vi "ConfigureRotatorPoint.vi"(10 "Rotator Position Min":dbl, 11 "Rotator Position Max":dbl) -> ()   [LabVIEW 2025]
doc: "Author: Scott Hannahs <sth@magnet.fsu.edu>\n\nThis software is licensed for use under the “MIT License\"\nCopyright (c) 2025 Scott Hannahs, sth@sth@magnet.sthnet.net\n\nPermission is hereby granted, free of charge, to any person obtaining a copy of this software and associated documentation files (the \"Software\"), to deal in the Software without restriction, including without limitation the rights to use, copy, modify, merge, publish, distribute, sublicense, and/or sell copies of the Software, and to permit persons to whom the Software is furnished to do so, subject to the following conditions: The above copyright notice and this permission notice shall be included in all copies or substantial portions of the Software.\n\nTHE SOFTWARE IS PROVIDED \"AS IS\", WITHOUT WARRANTY OF ANY KIND, EXPRESS OR IMPLIED, INCLUDING BUT NOT LIMITED TO THE WARRANTIES OF MERCHANTABILITY, FITNESS FOR A PARTICULAR PURPOSE AND NONINFRINGEMENT. IN NO EVENT SHALL THE AUTHORS OR COPYRIGHT HOLDERS BE LIABLE FOR ANY CLAIM, DAMAGES OR OTHER LIABILITY, WHETHER IN AN ACTION OF CONTRACT, TORT OR OTHERWISE, ARISING FROM, OUT OF OR IN CONNECTION WITH THE SOFTWARE OR THE USE OR OTHER DEALINGS IN THE SOFTWARE."
uses:
  Sub Controls/Instrument.ctl
  Sub Controls/NML GPIB List.ctl
panel:
  in  "Motor type":bool=TRUE
  out "Instrument":T1
  in  "Controls":refnum<vi>[](array[refnum])
  in  "GPIB Settings":T3 {"#16"."Parameters" format="%.3e"; "#20"."Parameters" format="%.3e"; "#18"."Parameters" format="%.3e"; "#17"."Parameters" format="%.3e"; "#19"."Parameters" format="%.3e"; "#11"."Parameters" format="%.3e"; "#15"."Parameters" format="%.3e"; "#13"."Parameters" format="%.3e"; "#12"."Parameters" format="%.3e"; "#14"."Parameters" format="%.3e"; "#6"."Parameters" format="%.3e"; "#10"."Parameters" format="%.3e"; "#8"."Parameters" format="%.3e"; "#7"."Parameters" format="%.3e"; "#9"."Parameters" format="%.3e"; "#1"."Parameters" format="%.3e"; "#5"."Parameters" format="%.3e"; "#3"."Parameters" format="%.3e"; "#2"."Parameters" format="%.3e"; "#4"."Parameters" format="%.3e"}
  in  "Done":bool
  # "BLM"
  # "IMS"
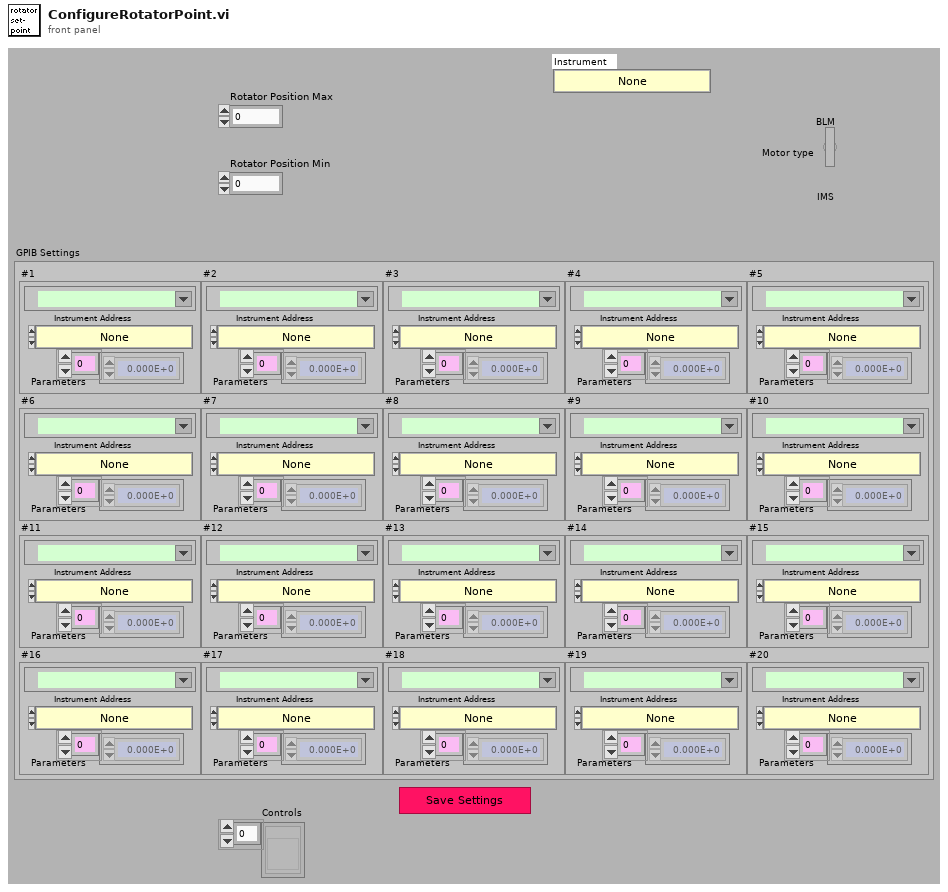
[diagram p1: front panel]
types:
  T1 = typedef "NML GPIB List.ctl" = enum16{"None", "Field", "Field - SCM1", "DMM", "DMM - HP 34401", "Keithley 2XXX", "Running DMM Ave", "Running HP34401", "Running K2XXX Ave", "SRS 830 - CH 1", "SRS 830 - CH1 & 2", "SRS PTC10", "Signal Rec 7265 - X", "Signal Rec 7265 - X&Y", "DRC 93C - Sample", "DRC 93C - Control", "DRC 93C - Sam&Con", "CryoCon Sensor A", "CryoCon Sensor B", "Cond 20C Sensor 1", "Cond 20C Sensor 2", "LS 336 Read", "LS 340 Read", "LS 370 Read", "LS 370 Select", "AVS 46 Bridge", "BLM Rotator Read Position", "Linear Research 700", "LR 700 Select", "Keithley 3330 - LCZ", "A-H Capacitance", "Digital Integrator", "SRS 400 Phot Ctr", "LakeShore VSM", "AMI He Level Meter", "Time Stamp", "Wait", "Invert Current", "K230 Linear V", "K230 VÅB^2", "Temp Ramp", "Power Ramp", "Freq Sweep", "LTC Stable T", "Scanner Step", "IMS Stepper Increment", "BLM Stepper Increment", "Omega CNi32"}
  T2 = typedef "Instrument.ctl" = cluster{"Instrument":T1, "Instrument Address":refnum<visa-resource-name>, "Parameters":dbl[]}
  T3 = cluster{"#1":T2, "#2":T2, "#3":T2, "#4":T2, "#5":T2, "#6":T2, "#7":T2, "#8":T2, "#9":T2, "#10":T2, "#11":T2, "#12":T2, "#13":T2, "#14":T2, "#15":T2, "#16":T2, "#17":T2, "#18":T2, "#19":T2, "#20":T2}
  T4 = cluster{"GPIB Settings[0]":T2, "GPIB Settings[1]":T2, "GPIB Settings[2]":T2, "GPIB Settings[3]":T2, "GPIB Settings[4]":T2, "GPIB Settings[5]":T2, "GPIB Settings[6]":T2, "GPIB Settings[7]":T2, "GPIB Settings[8]":T2, "GPIB Settings[9]":T2, "GPIB Settings[10]":T2, "GPIB Settings[11]":T2, "GPIB Settings[12]":T2, "GPIB Settings[13]":T2, "GPIB Settings[14]":T2, "GPIB Settings[15]":T2, "GPIB Settings[16]":T2, "GPIB Settings[17]":T2, "GPIB Settings[18]":T2, "GPIB Settings[19]":T2}
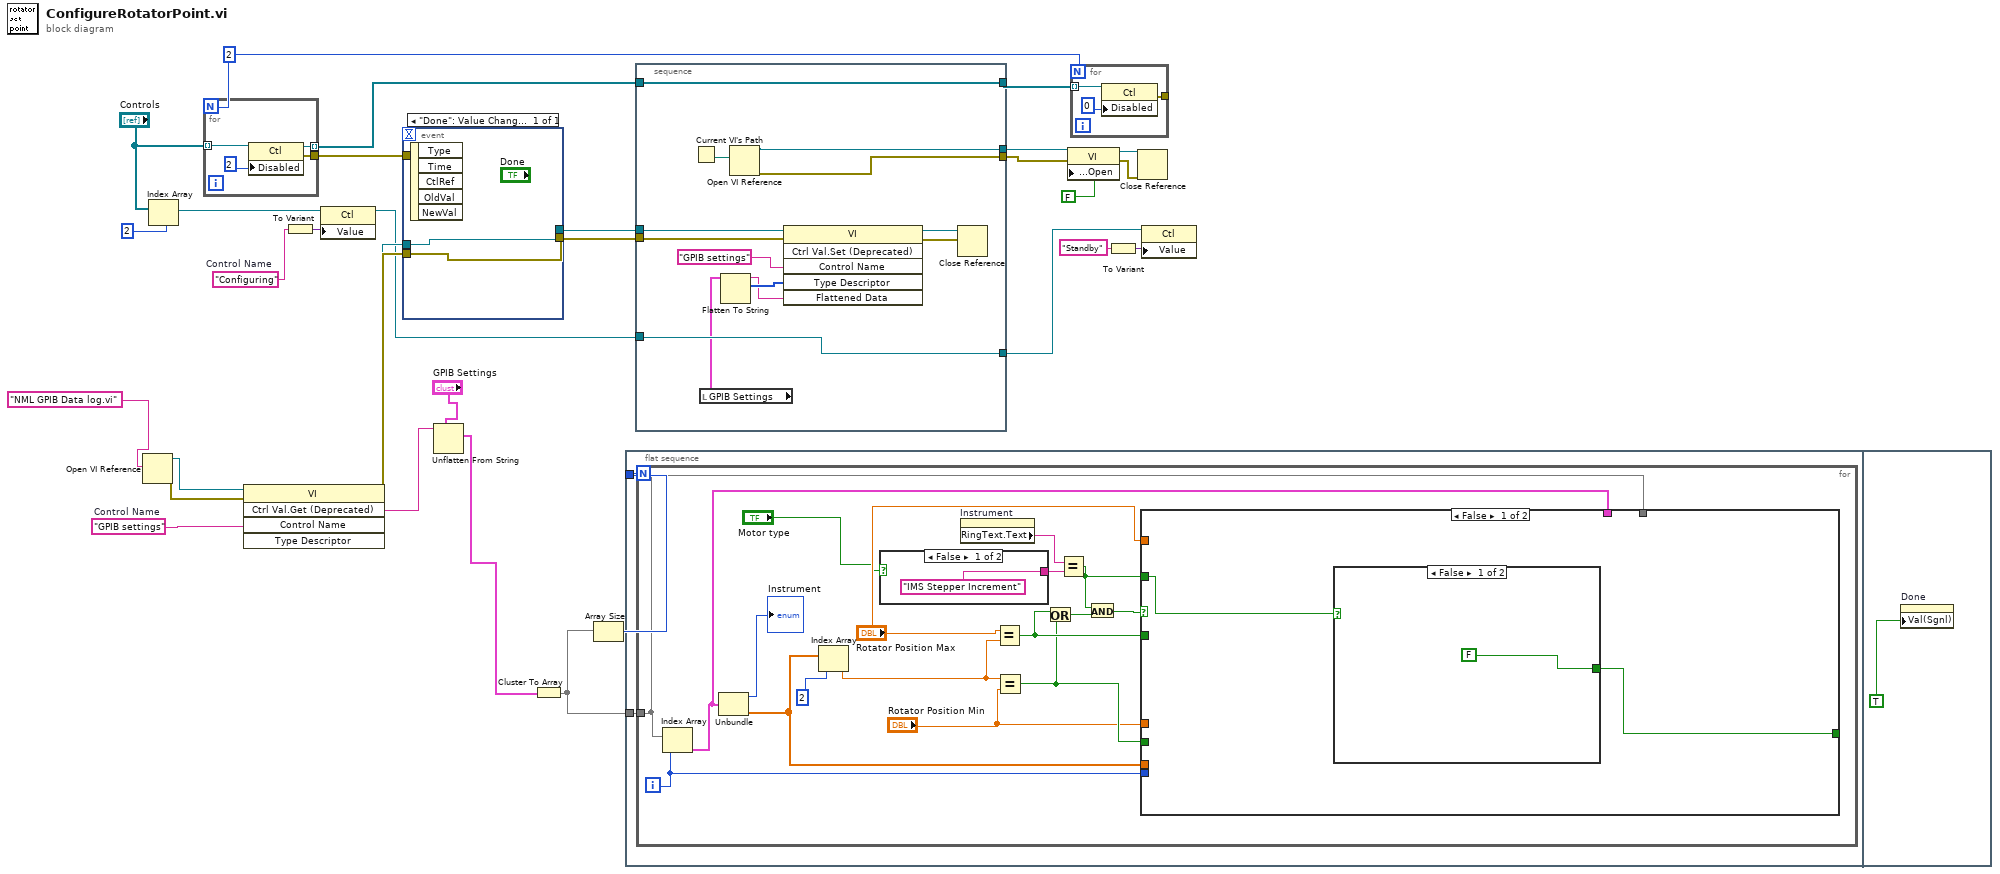
[diagram p0: block diagram]
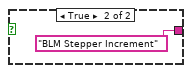
[diagram p2: hidden frame]
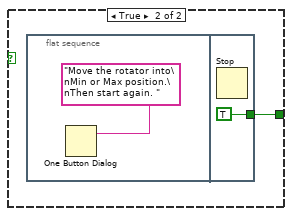
[diagram p3: hidden frame]
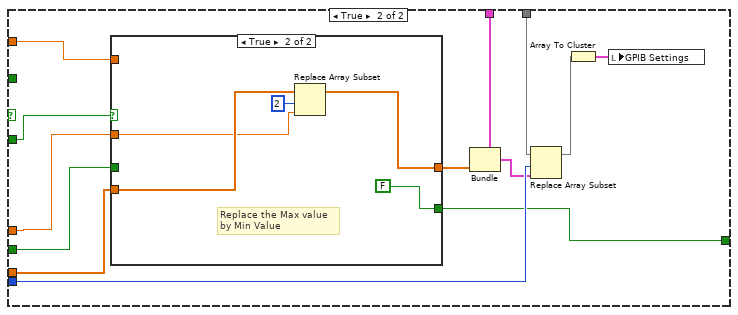
[diagram p4: hidden frame]
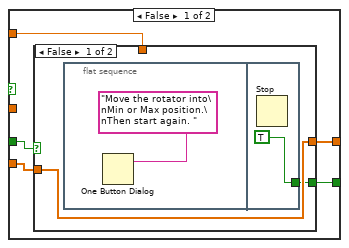
[diagram p5: hidden frame]
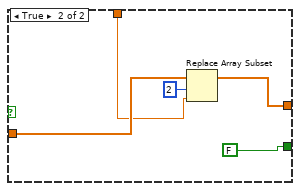
[diagram p6: hidden frame]
diagram:
  w15 = "Configuring"  # Control Name
  w18 = 2
  w30 = "GPIB settings"  # Control Name
  n1 = Open VI Reference(vi path="NML GPIB Data log.vi") -> (vi reference=w29:refnum<vi>, error out=w31:errorcluster)  [unwired: 5 in]
  n2 = Index Array(array="Controls", index=2) -> (element=w16:refnum<vi>)
  n3 = for {
    N: w18 -> [_]
    tunnel: "Controls" -> [w35] mode=indexing
    tunnel: [w33] -> w21
    tunnel: [w32] -> w20 mode=indexing
    n4 = property class="Ctl"(reference=w35, "Disabled"=u8 2) -> (reference out=w32:refnum<vi>, error out=w33:errorcluster)  [unwired: 1 in]
  }
  n5 = invoke class="VI" method="Ctrl Val.Get (Deprecated)"(reference=w29, error in=w31, "Control Name"=w30) -> (reference out=w9:refnum<vi>, error out=w24:errorcluster, "Get Control Value"=w27:string)  [unwired: 2 in, 2 out]
  n6 = To Variant(anything=w15) -> (Variant=w14:variant)
  n7 = property class="Ctl"(reference=w16, "Value"=w14) -> (reference out=w8:refnum<vi>)  [unwired: 1 in, 1 out]
  n8 = event shown="[0] \"Done\": Value Change" {
    selector: _ -> [_]
    dyn-events: _ -> [_]
    timeout: _ -> [_]
    tunnel: w9 -> [w37]
    tunnel: [w37] -> w26
    tunnel: [w36] -> w25
    tunnel: w24 -> [w36]
    tunnel: w21 -> [_]
    event "Done": Value Change {
      n9 = event-data() -> ()  [unwired: 1 in, 5 out]
    }
  }
  n10 = Unflatten From String(type="GPIB Settings", binary string=w27) -> (value=w5:T3)  [unwired: 3 in, 2 out]
  n11 = Cluster To Array(cluster=w5) -> (array=w6:T2[])
  n12 = Array Size(array=w6) -> (size(s)=w7:i32)
  n13 = flat-sequence {
    tunnel: w7 -> [w39]
    tunnel: w6 -> [w38]
    frame #0 {
      n14 = for {
        N: w39 -> [_]
        tunnel: w38 -> [w42]
        i -> [w41]
        n15 = Index Array(array=w42, index=w41) -> (element=w43:T2)
        n16 = Unbundle(w43) -> ("Instrument"=→"Instrument":T1, "Parameters"=w46:dbl[])  [unwired: 1 out]
        n17 = Index Array(array=w46, index=2) -> (element=w51:dbl)
        n18 = case shown="False" "Motor type" {
          tunnel: ["IMS Stepper Increment" ("y") "BLM Stepper Increment" ("y")] -> w54
          frame False {
          }
          frame True {
          }
        }
        n19 = property on="Instrument" class="Enum (strict)"() -> ("RingText.Text"=w55:string)  [unwired: 2 in, 2 out]
        n20 = Equal?(x="Rotator Position Max", y=w51) -> (x = y?=w49:bool)
        n21 = Equal?(x=w51, y="Rotator Position Min") -> (x = y?=w48:bool)
        n22 = Or(x=w49, y=w48) -> (x .or. y?=w52:bool)
        n23 = Equal?(x=w55, y=w54) -> (x = y?=w47:bool)
        n24 = And(x=w47, y=w52) -> (x .and. y?=w50:bool)
        n25 = case shown="False" w50 {
          tunnel: w49 -> [_ w77]
          tunnel: w48 -> [_ w73]
          tunnel: w47 -> [w60 _]
          tunnel: w46 -> [_ w76]
          tunnel: "Rotator Position Min" -> [_ w75]
          tunnel: "Rotator Position Max" -> [_ w74]
          tunnel: w43 -> [_ w71]
          tunnel: w42 -> [_ w70]
          tunnel: w41 -> [_ w69]
          tunnel: [w59 w67] -> _
          frame False {
            n26 = case shown="False" w60 {
              tunnel: [FALSE w62] -> w59
              frame False {
              }
              frame True {
                n27 = flat-sequence {
                  tunnel: [TRUE] -> w62
                  frame #0 {
                    n28 = One Button Dialog(message="Move the rotator into\nMin or Max position.\nThen start again. ") -> ()  [unwired: 1 in, 1 out]
                  }
                  frame #1 {
                    n29 = Stop() -> ()  [unwired: 1 in]
                  }
                }
              }
            }
          }
          frame True {
            n30 = case shown="True" w77 {
              tunnel: w76 -> [w82 w96]
              tunnel: w75 -> [_ w95]
              tunnel: w74 -> [w81 _]
              tunnel: w73 -> [w80 _]
              tunnel: [w79 w93] -> w72
              tunnel: [w78 FALSE] -> w67
              frame False {
                n31 = case shown="False" w80 {
                  tunnel: w82 -> [w84 w91]
                  tunnel: w81 -> [_ w90]
                  tunnel: [w84 w88] -> w79
                  tunnel: [w83 FALSE] -> w78
                  frame False {
                    n32 = flat-sequence {
                      tunnel: [TRUE] -> w83
                      frame #0 {
                        n33 = One Button Dialog(message="Move the rotator into\nMin or Max position.\nThen start again. ") -> ()  [unwired: 1 in, 1 out]
                      }
                      frame #1 {
                        n34 = Stop() -> ()  [unwired: 1 in]
                      }
                    }
                  }
                  frame True {
                    n35 = Replace Array Subset(array=w91, new element=w90, index=2) -> (w88:dbl[])
                  }
                }
              }
              frame True {
                # "Replace the Max value\nby Min Value"
                n36 = Replace Array Subset(array=w96, new element=w95, index=2) -> (w93:dbl[])
              }
            }
            n37 = Bundle(cluster=w71, "Parameters"=w72) -> (w68:T2)  [unwired: 2 in]
            n38 = Replace Array Subset(array=w70, new element=w68, index=w69) -> (w65:T2[])
            n39 = Array To Cluster(array=w65) -> (cluster=w66:T4)
            n40 = local write "GPIB Settings"(w66) -> ()
          }
        }
      }
    }
    frame #1 {
      n41 = property on="Done" class="Bool (strict)"("Val(Sgnl)"=TRUE ("Value (Signaling)")) -> ()  [unwired: 2 in, 2 out]
    }
  }
  n42 = stacked-sequence {
    tunnel: w26 -> [w104]
    tunnel: w25 -> [w103]
    tunnel: [w102] -> w23
    tunnel: [w101] -> w22
    tunnel: w20 -> [w100]
    tunnel: [w100] -> w12
    tunnel: [w99] -> w11
    tunnel: w8 -> [w99]
    frame #0 {
      n43 = Current VI's Path() -> (path=w105:path)
      n44 = local read "GPIB Settings"() -> (w98:T3)
      n45 = Flatten To String(anything=w98) -> (data string=w109:string, type string=w110:i16[])  [unwired: 3 in, 1 out]
      n46 = Open VI Reference(vi path=w105) -> (vi reference=w102:refnum<vi>, error out=w101:errorcluster)  [unwired: 5 in]
      n47 = invoke class="VI" method="Ctrl Val.Set (Deprecated)"(reference=w104, error in=w103, "Control Name"="GPIB settings", "Type Descriptor"=w110, "Flattened Data"=w109) -> (reference out=w107:refnum<vi>, error out=w106:errorcluster)  [unwired: 1 in, 4 out]
      n48 = Close Reference(reference=w107, error in (no error)=w106) -> ()  [unwired: 1 out]
    }
  }
  n49 = property class="VI"(reference=w23, error in=w22, "Front Panel Window:Open"=FALSE) -> (reference out=w2:refnum<vi>, error out=w3:errorcluster)
  n50 = for {
    N: w18 -> [_]
    tunnel: w12 -> [w113] mode=indexing
    tunnel: [w111] -> _
    n51 = property class="Ctl"(reference=w113, "Disabled"=u8 0) -> (error out=w111:errorcluster)  [unwired: 1 in, 1 out]
  }
  n52 = To Variant(anything="Standby" ("Control Name")) -> (Variant=w10:variant)
  n53 = Close Reference(reference=w2, error in (no error)=w3) -> ()  [unwired: 1 out]
  n54 = property class="Ctl"(reference=w11, "Value"=w10) -> ()  [unwired: 1 in, 2 out]
